vi "Aspect Ratio Score.vi"(8 "Equivalent Rect Short":dbl, 9 "Equivalent Rect Long":dbl, 10 "Height":dbl, 11 "Width":dbl) -> (2 "Horizontal":bool, 3 "Score":dbl)   [LabVIEW 2025]
doc: "Compare the ratio of the rectangle to that of the expected target. Score is in percent.\n\nSince inputs are particle measurements, the diagram doesn't expect to receive zero or negative values for either input."
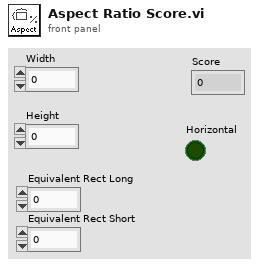
[diagram p1: front panel]
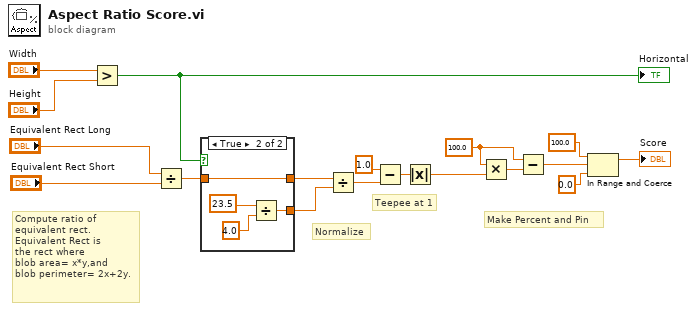
[diagram p0: block diagram]
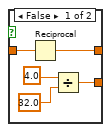
[diagram p2: hidden frame]
diagram:
  w8 = 100.0 ("x/y")
  # "Make Percent and Pin"
  # "Teepee at 1"
  # "Normalize"
  # "Compute ratio of\nequivalent rect.\nEquivalent Rect is\nthe rect where\nblob area= x*y,and\nblob perimeter= 2x+2y."
  n1 = Greater?(x="Width", y="Height") -> (0:w5:bool)
  "Horizontal" <- w5
  n2 = Divide(x="Equivalent Rect Long", y="Equivalent Rect Short") -> (x/y=w2:dbl)
  n3 = case shown="True" w5 {
    tunnel: w2 -> [w23 w27]
    tunnel: [w22 w27] -> w14
    tunnel: [w19 w24] -> w16
    frame False {
      n4 = Reciprocal(x=w23) -> (1/x=w22:dbl)
      n5 = Divide(x=4.0 ("y"), y=32.0) -> (x/y=w19:dbl)
    }
    frame True {
      n6 = Divide(x=23.5 ("y"), y=4.0) -> (x/y=w24:dbl)
    }
  }
  n7 = Divide(x=w14, y=w16) -> (x/y=w15:dbl)
  n8 = Subtract(x=1.0 ("y"), y=w15) -> (x-y=w10:dbl)
  n9 = Absolute Value(x=w10) -> (abs(x)=w7:dbl)
  n10 = Multiply(x=w8, y=w7) -> (x*y=w6:dbl)
  n11 = Subtract(x=w8, y=w6) -> (x-y=w11:dbl)
  n12 = In Range and Coerce(upper limit=100.0, x=w11, lower limit=0.0) -> (coerced(x)=→"Score":dbl)  [unwired: 1 out]
